vi "close TCP Client.vi"(8 "error in (no error)":errorcluster caption="错误输入（无错误）", 11 "LS-H600-TCP Client 输入":refnum<class "LS-H600-TCP Client.lvclass">) -> (0 "error out":errorcluster caption="错误输出", 3 "LS-H600-TCP Client 输出":refnum<class "LS-H600-TCP Client.lvclass">)   [LabVIEW 2022 SP3, in "LS-H600-TCP Client.lvlib" / "LS-H600-TCP Client.lvclass"]
uses:
  LS-H600-TCP Client.lvclass
  LS-H600-TCP Client.lvclass/LS-H600-TCP Client.ctl
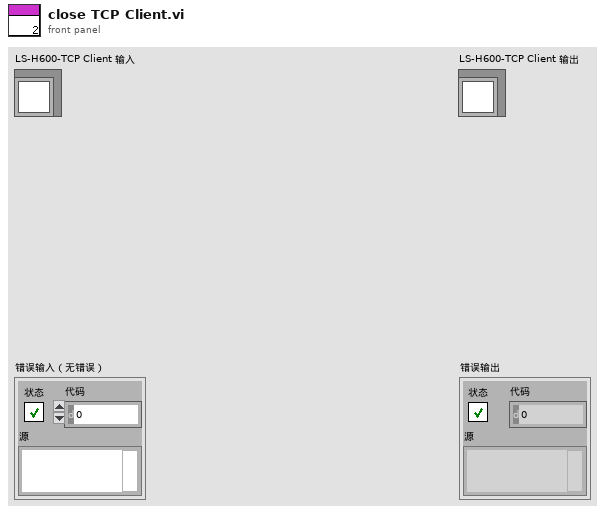
[diagram p1: front panel]
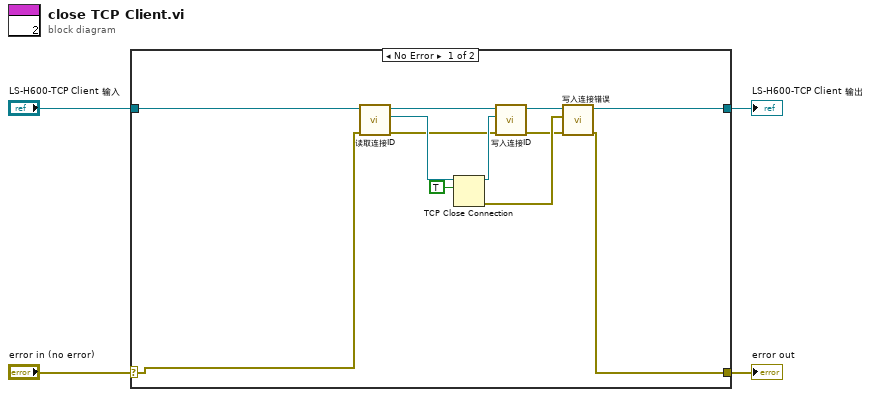
[diagram p0: block diagram]
diagram:
  n1 = case shown="No Error" "error in (no error)" {
    selector: "error in (no error)" -> [w15 w18]
    tunnel: [w11 w18] -> w3
    tunnel: [w13 w17] -> w1
    tunnel: "LS-H600-TCP Client 输入" -> [w16 w17]
    frame No Error {
      n2 = call "读取连接ID.vi"("error in (no error)"=w15, "LS-H600-TCP Client输入"=w16) -> ("error out"=w7:errorcluster, "连接ID"=w14:refnum<k5>, "LS-H600-TCP Client输出"=w10:refnum<class "LS-H600-TCP Client.lvclass">)  [unwired: 7 in]
      n3 = TCP Close Connection(connection ID=w14, abort (F)=TRUE ("中止(F)")) -> (connection ID out=w9:refnum<k5>, error out=w12:errorcluster)  [unwired: 1 in]
      n4 = call "写入连接ID.vi"("error in (no error)"=w7, "连接ID"=w9, "LS-H600-TCP Client输入"=w10) -> ("error out"=w6:errorcluster, "LS-H600-TCP Client输出"=w8:refnum<class "LS-H600-TCP Client.lvclass">)  [unwired: 7 in]
      n5 = call "写入连接错误.vi"("error in (no error)"=w6, "连接错误"=w12, "LS-H600-TCP Client输入"=w8) -> ("error out"=w11:errorcluster, "LS-H600-TCP Client输出"=w13:refnum<class "LS-H600-TCP Client.lvclass">)  [unwired: 7 in]
    }
    frame Error {
    }
  }
  "error out" <- w3
  "LS-H600-TCP Client 输出" <- w1
